vi "lp-server-timeouts.vi"() -> ()   [LabVIEW 2010]
uses:
  socket_type.ctl
  zmq_context.lvclass
  zeromq.lvlib
  zmq_socket.lvclass
panel:
  in  "stop?":bool
  out "loop":i32
  in  "timeout":u32=500
  in  "endpoint":string="tcp://127.0.0.1:5555"
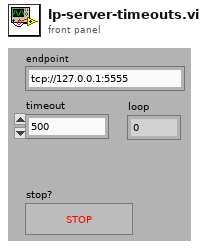
[diagram p1: front panel]
types:
  T1 = typedef "zeromq.lvlib/socket_type.ctl" = enum8{"ZMQ_PAIR", "ZMQ_PUB", "ZMQ_SUB", "ZMQ_REQ", "ZMQ_REP", "ZMQ_DEALER", "ZMQ_ROUTER", "ZMQ_PULL", "ZMQ_PUSH", "ZMQ_XPUB", "ZMQ_XSUB"}
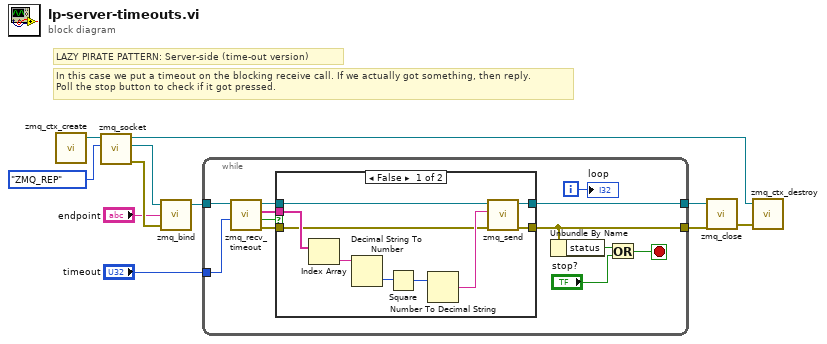
[diagram p0: block diagram]
diagram:
  # "In this case we put a timeout on the blocking receive call. If we actually got something, then reply.\nPoll the stop button to check if it got pressed."
  # "LAZY PIRATE PATTERN: Server-side (time-out version)"
  n1 = call "zmq_ctx_create.vi"() -> ("context out"=w6:refnum<class "zmq_context.lvclass">)  [unwired: 4 in, 1 out]
  n2 = call "zmq_socket.vi"("socket type"=socket_type."ZMQ_REP", "context in"=w6) -> ("error out"=w10:errorcluster, "socket out"=w2:refnum<class "zmq_socket.lvclass">, "context out"=w1:refnum<class "zmq_context.lvclass">)  [unwired: 3 in]
  n3 = call "zmq_bind.vi"("error in"=w10, "endpoint"="endpoint", "socket in"=w2) -> ("socket out"=w8:refnum<class "zmq_socket.lvclass">)  [unwired: 1 in, 1 out]
  n4 = while {
    tunnel: "timeout" -> [w21]
    tunnel: w8 -> [w23]
    tunnel: [w17] -> w5
    tunnel: [w16] -> w3
    i -> [w19]
    stop <- w13 stop-if-true
    n5 = call "zmq_recv_timeout.vi"("timeout (ms)"=w21, "socket in"=w23) -> ("error out"=w18:errorcluster, "timeout?"=w12:bool, "parts"=w20:string[], "socket out"=w22:refnum<class "zmq_socket.lvclass">)  [unwired: 2 in]
    n6 = case shown="False" w12 {
      tunnel: w22 -> [w32 w34]
      tunnel: w20 -> [w31 _]
      tunnel: w18 -> [w26 w33]
      tunnel: [w25 w34] -> w17
      tunnel: [w24 w33] -> w16
      frame False {
        n7 = Index Array(array=w31) -> (element=w30:string)  [unwired: 1 in]
        n8 = Decimal String To Number(string=w30) -> (number=w29:i32)  [unwired: 2 in, 1 out]
        n9 = Square(x=w29) -> (x^2=w28:i32)
        n10 = Number To Decimal String(number=w28) -> (decimal integer string=w27:string)  [unwired: 1 in]
        n11 = call "zmq_send.vi"("error in"=w26, "data"=w27, "socket in"=w32) -> ("error out"=w24:errorcluster, "socket out"=w25:refnum<class "zmq_socket.lvclass">)  [unwired: 4 in]
      }
      frame True {
      }
    }
    n12 = Unbundle By Name(w16) -> ("status"=w15:bool)
    n13 = Or(x=w15, y="stop?") -> (x .or. y?=w13:bool)
    "loop" <- w19
  }
  n14 = call "zmq_close.vi"("error in"=w3, "socket"=w5) -> ("error out"=w4:errorcluster)  [unwired: 3 in]
  n15 = call "zmq_ctx_destroy.vi"("error in"=w4, "context in"=w1) -> ()  [unwired: 3 in, 1 out]
